vi "Remove Zeros By Interpolation [DBL].vi"(8 "Error In":errorcluster, 11 "Array in":dbl[](array[numeric])) -> (0 "Error Out":errorcluster, 3 "Array out":dbl[](array[numeric]))   [LabVIEW 2021, in "Arrays.lvlib"]
doc: "Replaces zero elements by an interpolated value between the nearest elements or 1, whichever is largest.\nRepeats until there is no zero elements left or there is no change from one iteration to the next (in which case an error is returned)."
uses:
  Arrays.lvlib
  66d91d49-fe1b-45d2-a554-45b8f907f5ab.vi
  1162f6cf-722d-42c0-bbf8-002c29922fe6.vi
  <userlib>/_OpenG.lib/array/array.llb/Search 1D Array (DBL)__ogtk.vi
  Signed Array Index.vi
  <userlib>/_OpenG.lib/array/array.llb/openg_array.lvlib
  <vilib>/ErrorRing/Error Ring.xnode
  <vilib>/Utility/error.llb/Error Cluster From Error Code.vi
  Math/Math.lvlib
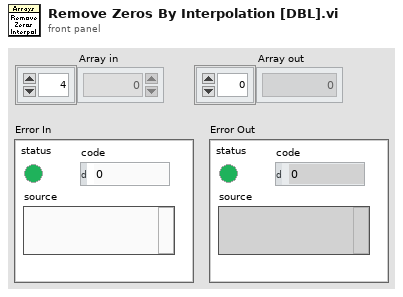
[diagram p1: front panel]
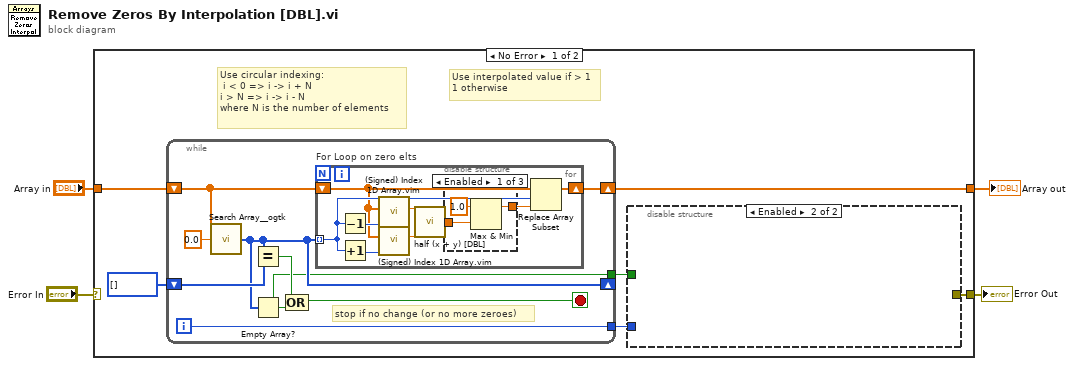
[diagram p0: block diagram]
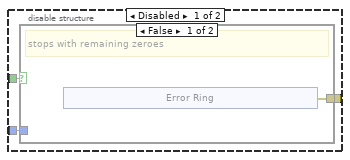
[diagram p2: hidden frame]
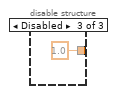
[diagram p5: hidden frame]
diagram:
  n1 = case shown="No Error" "Error In" {
    selector: "Error In" -> [_ w43]
    tunnel: "Array in" -> [w9 w42]
    tunnel: [w10 w43] -> w3
    tunnel: [w8 w42] -> w1
    frame No Error {
      # "Use interpolated value if > 1\n1 otherwise"
      # "Use circular indexing:\n i < 0 => i -> i + N\ni > N => i -> i - N\nwhere N is the number of elements"
      n2 = while {
        shift-right: [w25] -> w8
        shift-left: w9 -> [w26]
        shift-right: [w21] -> _
        shift-left: i32[] [] ("Indices of Elements") -> [w24]
        tunnel: [w19] -> w7
        tunnel: [w20] -> w5
        i -> [w20]
        stop <- w23 stop-if-true
        # "stop if no change (or no more zeroes)"
        n3 = call-poly <userlib>:"Search Array__ogtk.vi"("Array"=w26, "Element Data"=0.0) -> ("Indices of Elements"=w21:i32[])  [unwired: 7 in]
        n4 = Equal?(x=w21, y=w24) -> (x = y?=w22:bool)
        n5 = Empty Array?(array=w21) -> (empty?=w19:bool)
        n6 = Compound Arithmetic op=OR(w22, w19) -> (w23:bool)
        n7 = for "For Loop on zero elts" {
          tunnel: w21 -> [w35] mode=indexing
          shift-right: [w34] -> w25
          shift-left: w26 -> [w32]
          n8 = Decrement(x=w35) -> (x-1=w33:i32)
          n9 = Increment(x=w35) -> (x+1=w31:i32)
          n10 = call "(Signed) Index 1D Array.vim"("Signed Index"=w33, "Array"=w32) -> ("Array Element"=w30:dbl)  [unwired: 9 in]
          n11 = call "(Signed) Index 1D Array.vim"("Signed Index"=w31, "Array"=w32) -> ("Array Element"=w29:dbl)  [unwired: 9 in]
          n12 = call "half (x + y) [DBL].vi"("y"=w29, "x"=w30) -> ("(x+y)/2"=w36:dbl)  [unwired: 4 in]
          n13 = disable-structure shown="Enabled" {
            disable-tunnel: w36 -> [w39 w40 _]
            disable-tunnel: [w37 w40 1.0 ("(x+y)/2")] -> w28
            frame Enabled {
              n14 = Max & Min(x=1.0, y=w39) -> (max(x,y)=w37:dbl)  [unwired: 1 out]
            }
            frame Disabled {
            }
            frame Disabled {
            }
          }
          n15 = Replace Array Subset(array=w32, new element=w28, index=w35) -> (w34:dbl[])
        }
      }
      n16 = disable-structure shown="Enabled" {
        disable-tunnel: [w13 _] -> w10
        disable-tunnel: w7 -> [w12 _]
        disable-tunnel: w5 -> [w11 _]
        frame Disabled {
          n17 = case shown="False" w12 {
            tunnel: [w14 _] -> w13
            tunnel: w11 -> [_ _]
            frame False {
              # "stops with remaining zeroes"
              n18 = xnode "Error Ring"() -> ("error out"=w14:errorcluster)
            }
            frame True {
              # "no more zeroes"
            }
          }
        }
        frame Enabled {
        }
      }
    }
    frame Error {
    }
  }
  "Error Out" <- w3
  "Array out" <- w1
